vi "limit1 (SubVI).vi"(9 "default":cluster{"x dim":dbl, "y dim":dbl}, 10 "dim":cluster{"x dim":dbl, "y dim":dbl}, 11 "newVal":cluster{"x start":i32, "y start":i32}) -> (2 "curCoord":cluster{"x start":i32, "y start":i32})   [LabVIEW 2011]
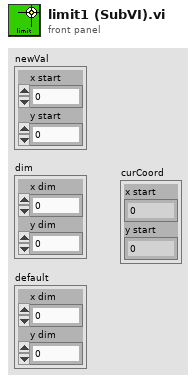
[diagram p1: front panel]
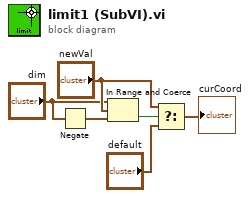
[diagram p0: block diagram]
diagram:
  n1 = Negate(x="dim") -> (-x=w5:cluster{"x dim":dbl, "y dim":dbl})
  n2 = In Range and Coerce(upper limit="dim", x="newVal", lower limit=w5) -> (In Range?=w3:bool)  [unwired: 1 out]
  n3 = Select(t="newVal", s=w3, f="default") -> (s? t:f=→"curCoord":cluster{"x dim":dbl, "y dim":dbl})
